vi "get_libraryBlacklist_p.vi"(0 "MoAgSy_Host":refnum<class "MoAgSy_Host.lvclass">, 5 "error in (no error)":errorcluster) -> (14 "dup MoAgSy_Host":refnum<class "MoAgSy_Host.lvclass">, 16 "Library Blacklist":string[](array[string]), 19 "error out":errorcluster)   [LabVIEW 2009, in "MoAgSy.lvlib" / "MoAgSy_Host.lvclass"]
doc: "<B>protected</B> VI returns blacklisted libraries of mobile agent host class.\nIs called by public get library Blacklist VI\n\nF.Berck@gsi.de\nGSI Darmstadt 2009"
uses:
  MoAgSy_Host.lvclass
  MoAgSy_Host.lvclass/MoAgSy_Host.ctl
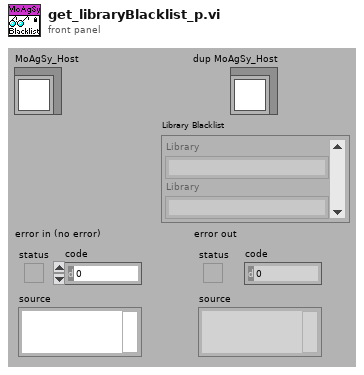
[diagram p1: front panel]
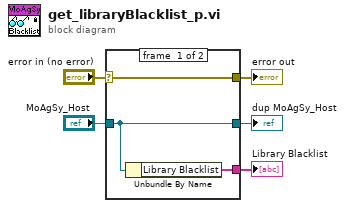
[diagram p0: block diagram]
diagram:
  n1 = case shown="No Error" "error in (no error)" {
    selector: "error in (no error)" -> [w8 w9]
    tunnel: [w8 w9] -> w4
    tunnel: [w7 w10] -> w2
    tunnel: "MoAgSy_Host" -> [w7 w10]
    tunnel: [w6 _] -> w1
    frame #0 {
      n2 = Unbundle By Name(w7) -> ("Library Blacklist"=w6:string[])
    }
    frame #1 {
    }
  }
  "error out" <- w4
  "dup MoAgSy_Host" <- w2
  "Library Blacklist" <- w1
